vi "Set AD Control Register.vi"(8 "error in (no error)":errorcluster, 11 "LINX-ADS1256 in":refnum<class "LINX-ADS1256.lvclass">) -> (0 "error out":errorcluster, 3 "LINX-ADS1256 out":refnum<class "LINX-ADS1256.lvclass">)   [LabVIEW 2020, in "LINX-ADS1256.lvclass"]
uses:
  LINX-ADS1256.lvclass
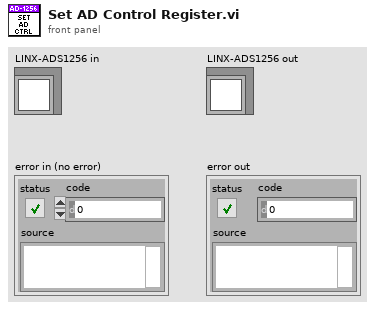
[diagram p1: front panel]
types:
  T1 = typedef "LINX-ADS1256.lvclass/Programmable Gain Selection.ctl" = enum16{"+/-5V (1)", "+/-2.5V (2)", "+/-1.25V (4)", "+/-0.625V (8)", "+/-312.5mV (16)", "+/-156.25mV (32)", "+/-78.125mV (64)"}
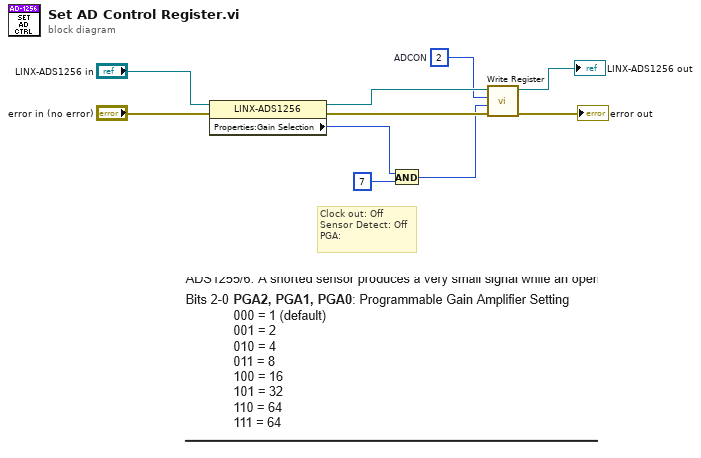
[diagram p0: block diagram]
diagram:
  w5 = u8 2  # ADCON
  # "Clock out: Off\nSensor Detect: Off\nPGA:"
  n1 = property class="LINX-ADS1256"(reference="LINX-ADS1256 in", error in="error in (no error)") -> (reference out=w7:refnum<class "LINX-ADS1256.lvclass">, error out=w8:errorcluster, "Properties:Gain Selection"=w3:T1)
  n2 = And(x=w3, y=u8 7 ("Data")) -> (x .and. y?=w1:u16)
  n3 = call "Write Register.vi"("error in (no error)"=w8, "Data"=w1, "Register Address"=w5, "LINX-ADS1256 in"=w7) -> ("error out"=→"error out":errorcluster, "LINX-ADS1256 out"=→"LINX-ADS1256 out":refnum<class "LINX-ADS1256.lvclass">)  [unwired: 6 in]
